vi "AI Waveform to Data UI.vi"(11 "AI dataout":waveform(dbl)[](array[waveform])) -> (2 "wf":waveform(dbl)[](array[waveform]), 3 "data":dbl[](array[numeric]))   [LabVIEW 2022 SP3]
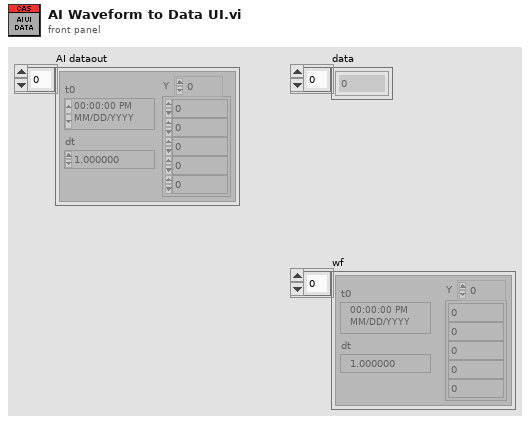
[diagram p1: front panel]
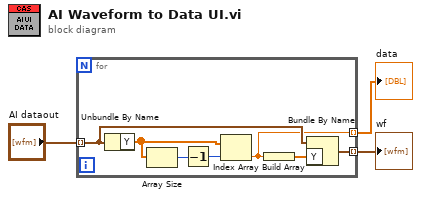
[diagram p0: block diagram]
diagram:
  n1 = for {
    tunnel: "AI dataout" -> [w10] mode=indexing
    tunnel: [w7] -> w1 mode=indexing
    tunnel: [w9] -> w3 mode=indexing
    n2 = Unbundle By Name(w10) -> ("Y"=w5:dbl[])
    n3 = Array Size(array=w5) -> (size(s)=w6:i32)
    n4 = Decrement(x=w6) -> (x-1=w4:i32)
    n5 = Index Array(array=w5, index=w4) -> (element=w7:dbl)
    n6 = Build Array(w7) -> (w8:dbl[])
    n7 = Bundle By Name(cluster=w10, "Y"=w8) -> (w9:waveform(dbl))
  }
  "wf" <- w3
  "data" <- w1
